vi "LV86_Kernel.vi"(2 "Kernel":sgl[][](array[numeric])=[[1.0, 1.0, 1.0], [1.0, 1.0, 1.0], [1.0, 1.0, 1.0]] format="%.2f", 3 "Image in":T1 {"Dialogs" format="%.0b"}) -> (1 "Image out":T1 {"Dialogs" format="%.0b"})   [LabVIEW 2024]
doc: "This VI convolves a given kernel with the incoming image."
uses:
  <userlib>/ImageProcessing/QTLIB_2595_LV86/QT_Image.ctl
  <vilib>/Analysis/2dsp.llb/2D Convolution (DBL).vi
  <vilib>/Analysis/NI_AALPro.lvlib
panel:
  # "This VI convolves a given kernel with the incoming image."
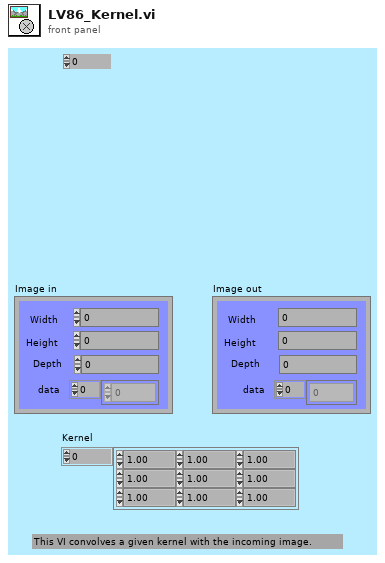
[diagram p1: front panel]
types:
  T1 = typedef "QT_Image.ctl" = cluster{"Width":i32, "Height":i32, "Depth":i32, "data":u8[], "Compressed data":u8[], "Color table":u32[], "Duration":i32, "Options":i32, "Timestamp":i32, "ID":i32, "Reserved":i32, "Dialogs":u32}
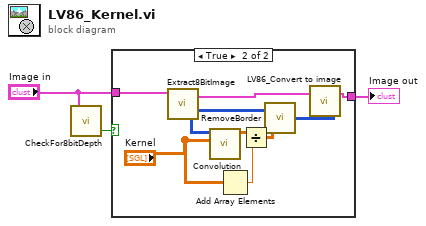
[diagram p0: block diagram]
diagram:
  n1 = call <userlib>:"CheckFor8bitDepth.vi"("Image in"="Image in") -> ("Success?"=w3:bool)  [unwired: 2 out]
  n2 = case shown="True" w3 {
    tunnel: "Image in" -> [w4 w10]
    tunnel: [w4 w8] -> w1
    frame False {
    }
    frame True {
      n3 = call <userlib>:"Extract8BitImage.vi"("Image in"=w10) -> ("Intensity Graph"=w6:u8[][], "Image out"=w9:T1)  [unwired: 1 in]
      n4 = call-poly <vilib>:"Convolution.vi"("Y"="Kernel", "X"=w6) -> ("X * Y"=w12:dbl[][])  [unwired: 2 in, 7 out]
      n5 = Add Array Elements(numeric array="Kernel") -> (sum=w13:sgl)
      n6 = Divide(x=w12, y=w13) -> (x/y=w7:dbl[][])
      n7 = call <userlib>:"RemoveBorder.vi"("Larger Image"=w7, "Original Image"=w6) -> ("Subset"=w5:u8[][])
      n8 = call <userlib>:"LV86_Convert to image.vi"("Intensity Graph"=w5, "Image In"=w9) -> ("Image Out"=w8:T1)  [unwired: 1 in]
    }
  }
  "Image out" <- w1
